vi "Read Config File.vi"(8 "Error In":errorcluster, 10 "Wash Options":string[](array[string]), 11 "File Path Control":path) -> (0 "Error Out":errorcluster, 2 "Wash Option Parameters":T1[](array[typedef]))   [LabVIEW 2018]
doc: "This VI is used to read wash parameters like station and time."
uses:
  Controls/Wash Option Parameters.ctl
  <vilib>/Utility/config.llb/Read Key (I32).vi
  <vilib>/Utility/config.llb/NI_LVConfig.lvlib
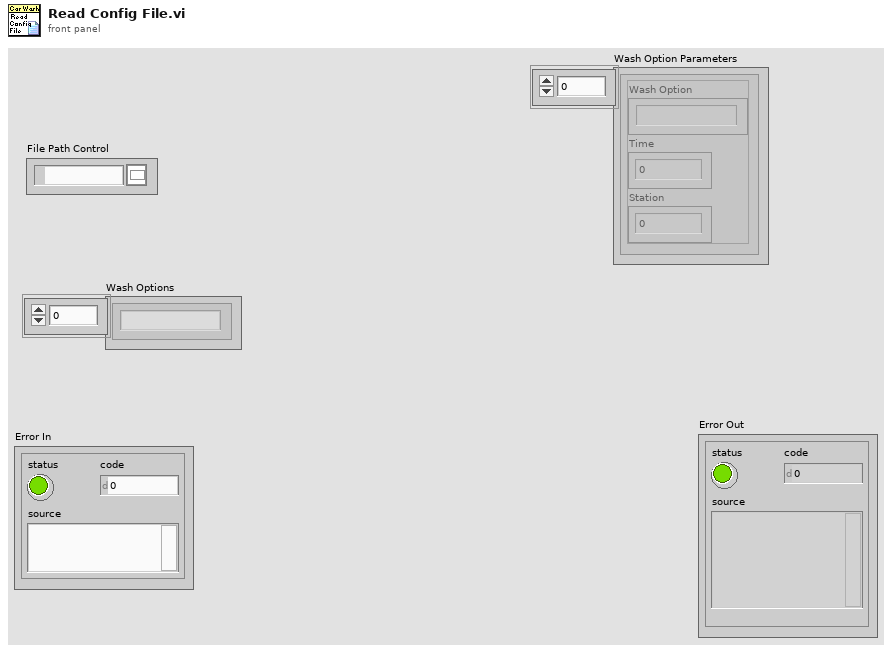
[diagram p1: front panel]
types:
  T1 = typedef "Wash Option Parameters.ctl" = cluster{"Wash Option":string, "Time":i32, "Station":i32}
  T2 = typedef "NI_LVConfig.lvlib/Config Data RefNum.ctl" = refnum<k1>
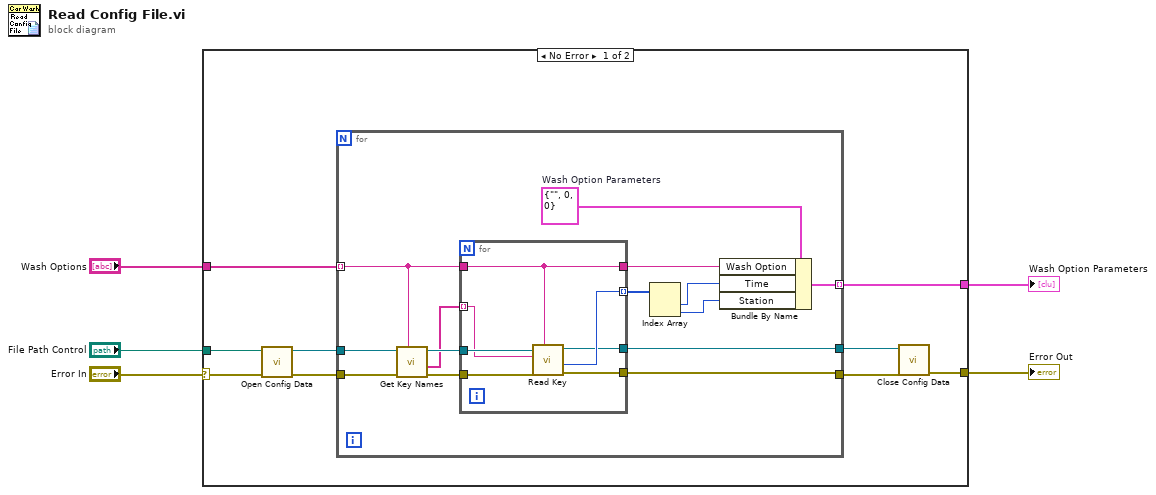
[diagram p0: block diagram]
diagram:
  n1 = case shown="No Error" "Error In" {
    selector: "Error In" -> [w13 w36]
    tunnel: [w6 w36] -> w4
    tunnel: "File Path Control" -> [w14 _]
    tunnel: "Wash Options" -> [w10 _]
    tunnel: [w9 _] -> w1
    frame No Error {
      n2 = call <vilib>:"Open Config Data.vi"("error in (no error)"=w13, "configuration file path"=w14) -> ("error out"=w12:errorcluster, "refnum"=w11:T2)  [unwired: 7 in, 1 out]
      n3 = for {
        tunnel: w11 -> [w24]
        tunnel: w10 -> [w22] mode=indexing
        tunnel: [w16] -> w9 mode=indexing
        tunnel: [w15] -> w7
        tunnel: w12 -> [w27]
        tunnel: [w28] -> w8
        w21 = T1 {"Wash Option"="", "Time"=0, "Station"=0}  # Wash Option Parameters
        n4 = call <vilib>:"Get Key Names.vi"("section"=w22, "error in (no error)"=w27, "refnum"=w24) -> ("error out"=w26:errorcluster, "key names"=w23:string[], "refnum out"=w25:T2)  [unwired: 5 in, 1 out]
        n5 = for {
          tunnel: w26 -> [w35]
          tunnel: w25 -> [w34]
          tunnel: [w33] -> w28
          tunnel: w23 -> [w32] mode=indexing
          tunnel: w22 -> [w31]
          tunnel: [w31] -> w20
          tunnel: [w30] -> w19 mode=indexing
          tunnel: [w29] -> w15
          n6 = call-poly <vilib>:"Read Key.vi"("section"=w31, "error in (no error)"=w35, "key"=w32, "refnum"=w34) -> ("error out"=w33:errorcluster, "value"=w30:i32, "refnum out"=w29:T2)  [unwired: 4 in, 1 out]
        }
        n7 = Index Array(array=w19) -> (element #1=w18:i32, element #2=w17:i32)  [unwired: 2 in]
        n8 = Bundle By Name(cluster=w21, "Wash Option"=w20, "Time"=w18, "Station"=w17) -> (w16:T1)
      }
      n9 = call <vilib>:"Close Config Data.vi"("error in (no error)"=w8, "refnum"=w7) -> ("error out"=w6:errorcluster)  [unwired: 8 in, 1 out]
    }
    frame Error {
    }
  }
  "Error Out" <- w4
  "Wash Option Parameters" <- w1
